vi "Interrupt Test.vi"() -> ()   [LabVIEW 2011, in "Diamond Universal Driver.lvlib"]
uses:
  Diamond Universal Driver.lvlib
  constants.vi
  Controls/board type.ctl
  Controls/dscBool.ctl
  Controls/dsccb.ctl
  support/dlls/mm32at.dll
  IO/DSCS.ctl
panel:
  in  "milliseconds to wait":u32
  out "status":T1 {"analog" items=["FALSE", "TRUE"]; "op_type" format="%.0x"}
  out "dsccbOut":T3 {"RMM DAC 4_7 ext en" items=["FALSE", "TRUE"]; "RMM DAC 0_3 ext en" items=["FALSE", "TRUE"]; "RMM mode 16bit" items=["FALSE", "TRUE"]; "RMM external trig c3" items=["FALSE", "TRUE"]; "RMM external trig" items=["FALSE", "TRUE"]; "base addr" format="%x"; "board type" items=["DMM16"=0, "RMM"=1, "TMM"=2, "OPMM"=3, "DMM"=4, "SMM"=5, "GMM"=6, "QMM"=7, "ZMM"=8, "PMM"=9, "OMM"=10, "RMM416"=11, "DMM32AT"=12, "EMMDIO"=13, "RMM1612"=14, "DMMAT"=15, "DMM16AT"=16, "IR104"=17, "EMM8"=18, "PROM"=19, "HERCEBX"=20, "CPT"=21, "DMM48AT"=22, "OMMIO"=23, "DIO82C55"=24, "ATHENA"=25, "METIS"=26, "DMM32XAT"=27, "ELEKTRA"=28, "GPIO11_9513"=29, "GPIO11_DIO"=30, "GPIO21"=31, "PSD"=32, "ATHENAII"=33, "DMM32DXAT"=34, "HELIOS"=35, "NEPTUNE"=36, "TEST"=126, "RAW"=127, "DRVR"=255]}
  out "error out 3":errorcluster
  in  "Boolean":bool
  out "Interrupts":u32
  out "error out":errorcluster
  out "error":u8
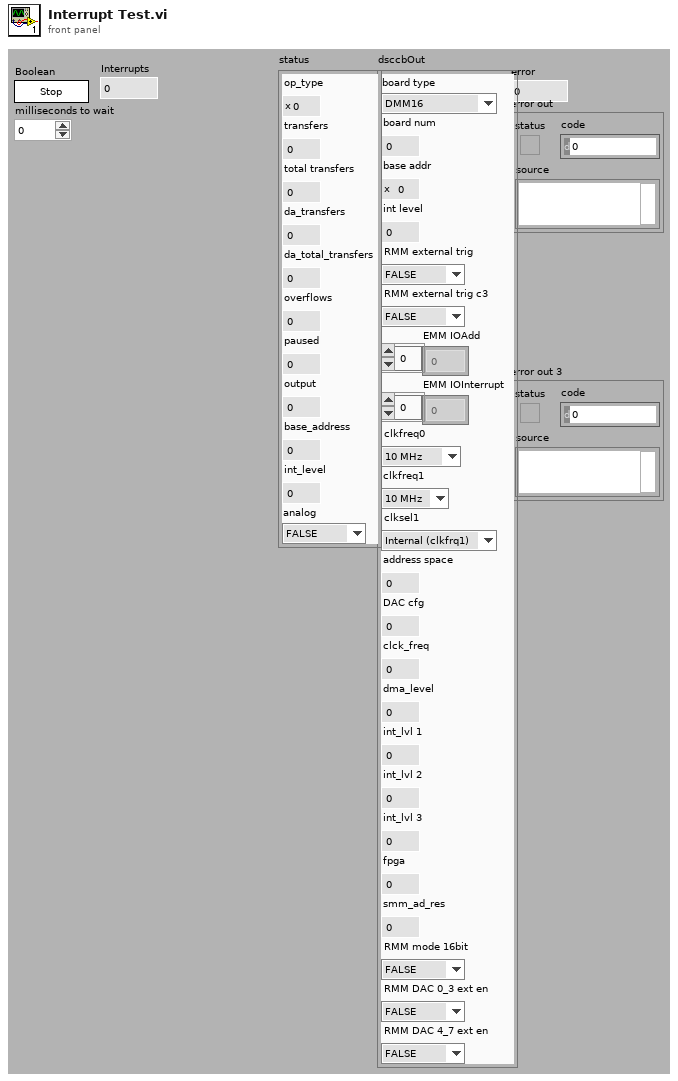
[diagram p1: front panel]
types:
  T1 = typedef "Diamond Universal Driver.lvlib/DSCS.ctl" = cluster{"op_type":u8, "transfers":u32, "total transfers":u32, "da_transfers":u32, "da_total_transfers":u32, "overflows":u32, "paused":u8, "output":u8, "base_address":u16, "int_level":u8, "analog":T2}
  T2 = typedef "dscBool.ctl" = i32
  T3 = typedef "dsccb.ctl" = cluster{"board type":T4, "board num":i16, "base addr":u16, "int level":u8, "RMM external trig":T2, "RMM external trig c3":T2, "EMM IOAdd":u16[], "EMM IOInterrupt":u16[], "clkfreq0":enum8{"10 MHz", "1 MHz"}, "clkfreq1":enum8{"10 MHz", "1 MHz"}, "clksel1":enum8{"Internal (clkfrq1)", "External"}, "address space":dbl, "DAC cfg":u8, "clck_freq":i32, "dma_level":u8, "int_lvl 1":u8, "int_lvl 2":u8, "int_lvl 3":u8, "fpga":u16, "smm_ad_res":u8, "RMM mode 16bit":T2, "RMM DAC 0_3 ext en":T2, "RMM DAC 4_7 ext en":T2}
  T4 = typedef "board type.ctl" = u8
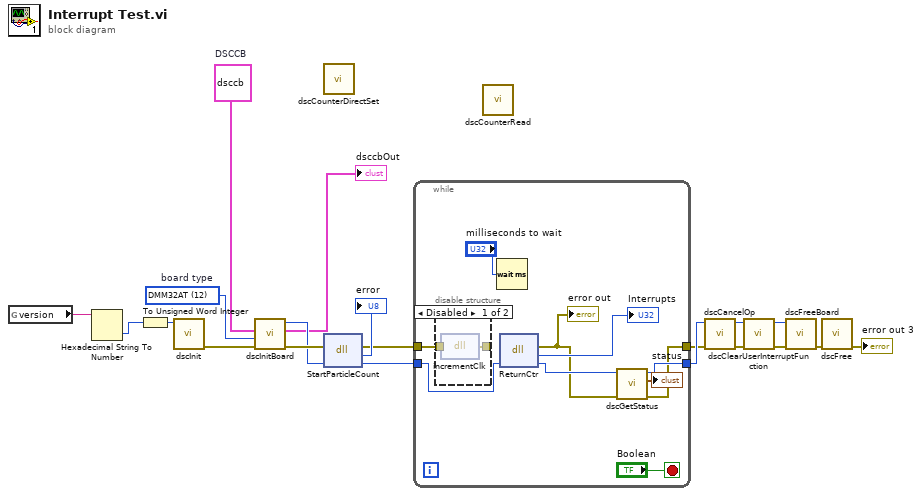
[diagram p0: block diagram]
diagram:
  w15 = T3 {"board type"=12, "board num"=1, "base addr"=768, "int level"=3, "RMM external trig"=0, "RMM external trig c3"=0, "EMM IOAdd"=[0, 0, 0, 0, 0, 0, 0, 0], "EMM IOInterrupt"=[0, 0, 0, 0, 0, 0, 0, 0], "clkfreq0"=enum."10 MHz", "clkfreq1"=enum."10 MHz", "clksel1"=enum."Internal (clkfrq1)", "address space"=0.0, "DAC cfg"=0, "clck_freq"=0, "dma_level"=0, "int_lvl 1"=0, "int_lvl 2"=0, "int_lvl 3"=0, "fpga"=0, "smm_ad_res"=0, "RMM mode 16bit"=0, "RMM DAC 0_3 ext en"=0, "RMM DAC 4_7 ext en"=0}  # DSCCB
  w16 = T4 12 items=["DMM16"=0, "RMM"=1, "TMM"=2, "OPMM"=3, "DMM"=4, "SMM"=5, "GMM"=6, "QMM"=7, "ZMM"=8, "PMM"=9, "OMM"=10, "RMM416"=11, "DMM32AT"=12, "EMMDIO"=13, "RMM1612"=14, "DMMAT"=15, "DMM16AT"=16, "IR104"=17, "EMM8"=18, "PROM"=19, "HERCEBX"=20, "CPT"=21, "DMM48AT"=22, "OMMIO"=23, "DIO82C55"=24, "ATHENA"=25, "METIS"=26, "DMM32XAT"=27, "ELEKTRA"=28, "GPIO11_9513"=29, "GPIO11_DIO"=30, "GPIO21"=31, "PSD"=32, "ATHENAII"=33, "DMM32DXAT"=34, "HELIOS"=35, "NEPTUNE"=36, "TEST"=126, "RAW"=127, "DRVR"=255]  # board type
  n1 = global read "constants.vi" "version"() -> (w20:string)
  n2 = Hexadecimal String To Number(string=w20) -> (number=w18:u32)  [unwired: 2 in, 1 out]
  n3 = To Unsigned Word Integer(number=w18) -> (unsigned 16bit integer=w19:u16)
  n4 = call "dscInit.vi"("versionIn"=w19) -> ("error out"=w17:errorcluster)  [unwired: 9 in, 1 out]
  n5 = call "dscInitBoard.vi"("error in"=w17, "board type"=w16, "DSCCB"=w15) -> ("error out"=w3:errorcluster, "dsccbOut"=→"dsccbOut":T3, "boardHandleOut"=w2:i16)  [unwired: 6 in]
  n6 = call "dscCounterDirectSet.vi"() -> ()  [unwired: 10 in, 2 out]
  n7 = dll-call lib="C:/Users/mrichardson/Documents/Web Based Version Control SW/Reusable/Diamond Universal Driver/support/dlls/mm32at.dll" fn="StartParticleCount"(error in=w3, "board"=w2) -> (error out=w13:errorcluster, "error"=→"error":u8, "board"=w12:i16)  [unwired: 2 in, 1 out]
  n8 = while {
    tunnel: w13 -> [w22]
    tunnel: w12 -> [w21]
    tunnel: [w26] -> w6
    tunnel: [w24] -> w5
    stop <- "Boolean" stop-if-true
    n9 = disable-structure shown="Disabled" {
      disable-tunnel: [w32 w33] -> _
      disable-tunnel: w22 -> [w31 w33]
      frame Disabled {
        n10 = dll-call lib="C:/Users/mrichardson/Documents/Web Based Version Control SW/Reusable/Diamond Universal Driver/support/dlls/mm32at.dll" fn="incrementClk"(error in=w31) -> (error out=w32:errorcluster)  [unwired: 3 in, 1 out]
      }
      frame Enabled {
      }
    }
    n11 = Wait (ms)(milliseconds to wait="milliseconds to wait") -> ()  [unwired: 1 out]
    n12 = dll-call lib="C:/Users/mrichardson/Documents/Web Based Version Control SW/Reusable/Diamond Universal Driver/support/dlls/mm32at.dll" fn="ReturnCtr"("board"=w21) -> (error out=w25:errorcluster, "val"=→"Interrupts":u32, "board"=w27:i16)  [unwired: 3 in, 1 out]
    "error out" <- w25
    n13 = call "dscGetStatus.vi"("error in"=w25, "board"=w27) -> ("error out"=w24:errorcluster, "status"=→"status":T1, "boardOut"=w26:i16)  [unwired: 7 in]
  }
  n14 = call "dscCounterRead.vi"() -> ()  [unwired: 9 in, 3 out]
  n15 = call "dscCancelOp.vi"("error in"=w5, "board"=w6) -> ("error out"=w9:errorcluster, "boardOut"=w10:i16)  [unwired: 8 in]
  n16 = call "dscClearUserInterruptFunction.vi"("error in"=w9, "board"=w10) -> ("error out"=w7:errorcluster, "boardOut"=w8:i16)  [unwired: 8 in]
  n17 = call "dscFreeBoard.vi"("error in"=w7, "boardIn"=w8) -> ("error out"=w11:errorcluster)  [unwired: 8 in, 1 out]
  n18 = call "dscFree.vi"("error in"=w11) -> ("error out"=→"error out 3":errorcluster)  [unwired: 10 in]
